vi "SaveVIsettings.vi"(11 "path":path) -> ()   [LabVIEW 2011]
doc: "This VI saves the controls of the VI you specify in VI path to settings.dat using the Configuration File VIs."
uses:
  <vilib>/Utility/config.llb/Write Key (String).vi
  <vilib>/Utility/config.llb/NI_LVConfig.lvlib
panel:
  # "Select Help»Show Context Help and move the cursor over the VI icon to display help for this VI."
  # "Instructions:\n1. Enter the path to settings.dat in the Configuration File path field.\n2. Enter the path to a VI with controls in the VI path field.\n3. Run the VI."
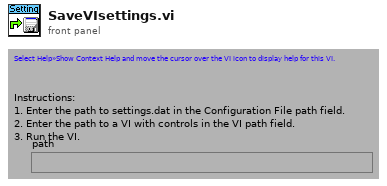
[diagram p1: front panel]
types:
  T1 = cluster{"name":string, "type desc":i16[], "flat data":string}[]
  T2 = typedef "NI_LVConfig.lvlib/Config Data RefNum.ctl" = refnum<k1>
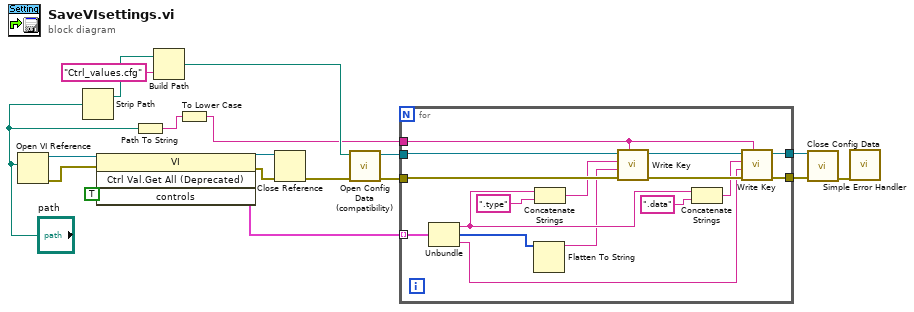
[diagram p0: block diagram]
diagram:
  n1 = Open VI Reference(vi path="path") -> (vi reference=w7:refnum<vi>, error out=w9:errorcluster)  [unwired: 5 in]
  n2 = Strip Path(path="path") -> (stripped path=w6:path)  [unwired: 1 out]
  n3 = invoke class="VI" method="Ctrl Val.Get All (Deprecated)"(reference=w7, error in=w9, "controls"=TRUE) -> (reference out=w11:refnum<vi>, error out=w12:errorcluster, "Get All Control Values"=w10:T1)  [unwired: 1 in, 1 out]
  n4 = Path To String(path="path") -> (string=w2:string)
  n5 = Build Path(base path=w6, name or relative path="Ctrl_values.cfg") -> (appended path=w4:path)
  n6 = To Lower Case(string=w2) -> (all lower case string=w1:string)
  n7 = Close Reference(reference=w11, error in (no error)=w12) -> (error out=w18:errorcluster)
  n8 = call <vilib>:"Open Config Data (compatibility).vi"("error in (no error)"=w18, "configuration file path"=w4) -> ("error out"=w14:errorcluster, "refnum"=w13:T2)  [unwired: 7 in, 1 out]
  n9 = for {
    tunnel: w10 -> [w34] mode=indexing
    tunnel: w1 -> [w22]
    tunnel: w13 -> [w33]
    tunnel: w14 -> [w32]
    tunnel: [w21] -> w15
    tunnel: [w20] -> w16
    n10 = Unbundle(w34) -> ("name"=w29:string, "type desc"=w27:i16[], "flat data"=w23:string)
    n11 = Flatten To String(anything=w27) -> (data string=w19:string)  [unwired: 3 in, 2 out]
    n12 = Concatenate Strings(w29, ".type" ("string")) -> (w28:string)
    n13 = call-poly <vilib>:"Write Key.vi"("section"=w22, "error in (no error)"=w32, "value"=w19, "key"=w28, "refnum"=w33) -> ("error out"=w25:errorcluster, "refnum out"=w26:T2)  [unwired: 4 in, 1 out]
    n14 = Concatenate Strings(w29, ".data" ("string")) -> (w24:string)
    n15 = call-poly <vilib>:"Write Key.vi"("section"=w22, "error in (no error)"=w25, "value"=w23, "key"=w24, "refnum"=w26) -> ("error out"=w20:errorcluster, "refnum out"=w21:T2)  [unwired: 4 in, 1 out]
  }
  n16 = call <vilib>:"Close Config Data.vi"("error in (no error)"=w16, "refnum"=w15) -> ("error out"=w17:errorcluster)  [unwired: 8 in, 1 out]
  n17 = call <vilib>:"Simple Error Handler.vi"("error in (no error)"=w17) -> ()  [unwired: 4 in, 5 out]
